vi "MATLAB.vi"(4 "Marker Style":string, 5 "Border Hit Style":string, 6 "Line Style":string, 7 "Border Win Color":u32, 8 "error in (no error)":errorcluster, 9 "Border Loss Color":u32, 10 "Ball Coordinates":cluster{"Array":dbl[], "Array 2":dbl[]}[](array[cluster]), 11 "Folder Path":path) -> (0 "error out":errorcluster, 3 "MATLAB Script":string)   [LabVIEW 2023]
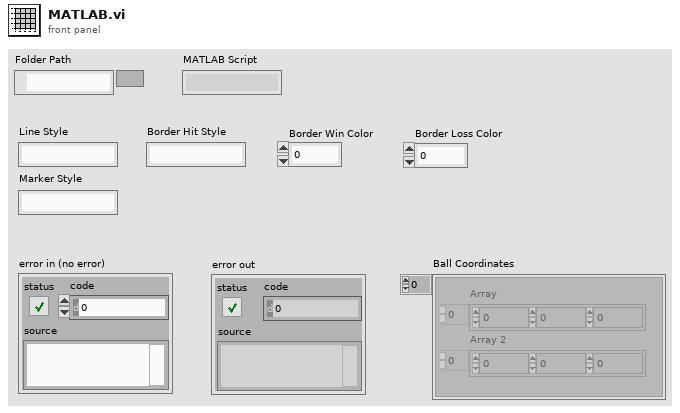
[diagram p1: front panel]
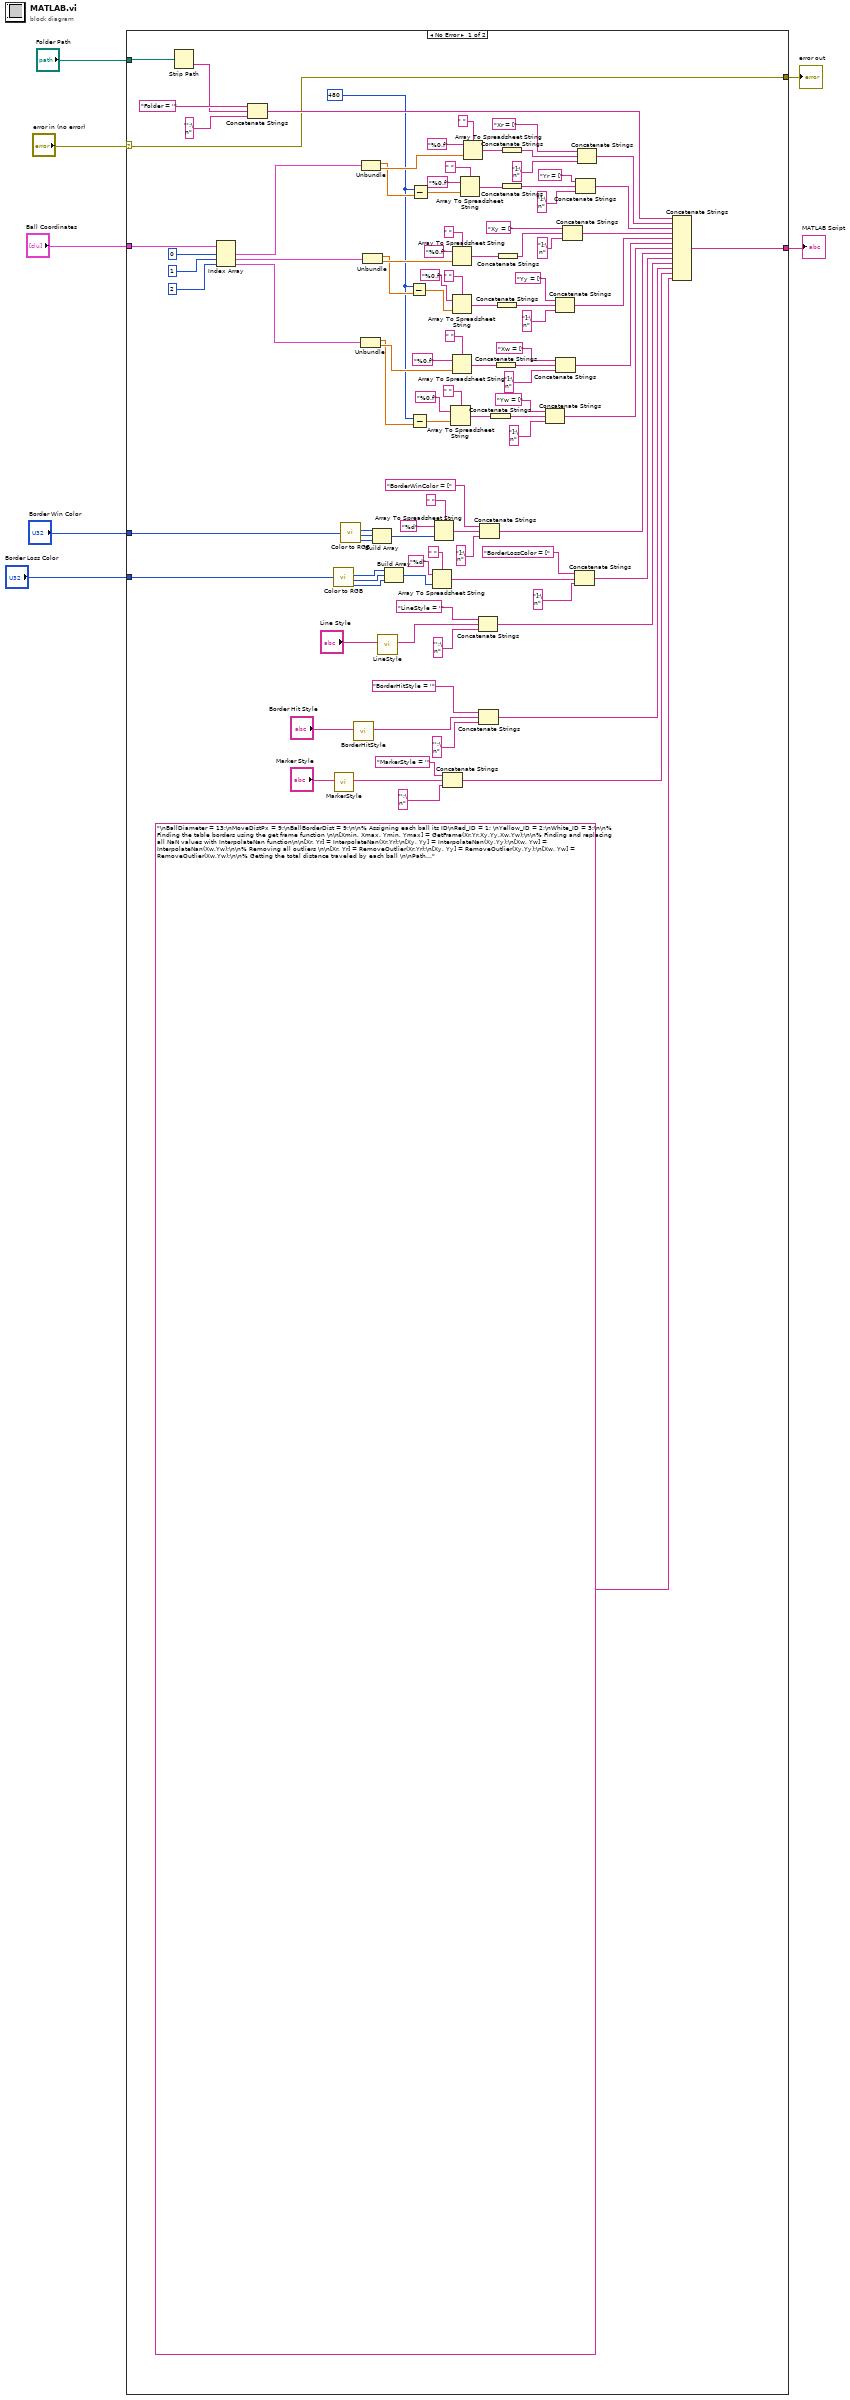
[diagram p0: block diagram]
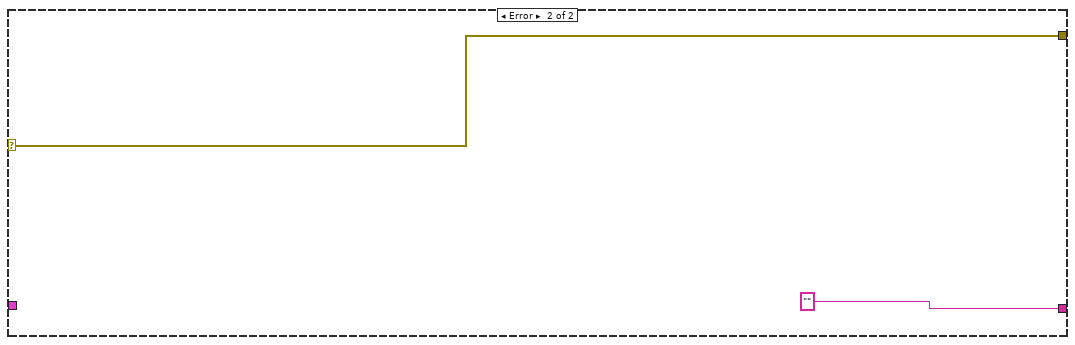
[diagram p2: hidden frame]
diagram:
  n1 = case shown="No Error" "error in (no error)" {
    selector: "error in (no error)" -> [w27 w113]
    tunnel: "Folder Path" -> [w111 _]
    tunnel: "Ball Coordinates" -> [w106 _]
    tunnel: "Border Win Color" -> [w48 _]
    tunnel: [w27 w113] -> w3
    tunnel: [w35 ""] -> w2
    tunnel: "Border Loss Color" -> [w26 _]
    frame No Error {
      w28 = 480
      n2 = Strip Path(path=w111) -> (name=w108:string)  [unwired: 1 out]
      n3 = Index Array(array=w106, index #1=0, index #2=1, index #3=2) -> (element #1=w102:cluster{"Array":dbl[], "Array 2":dbl[]}, element #2=w101:cluster{"Array":dbl[], "Array 2":dbl[]}, element #3=w100:cluster{"Array":dbl[], "Array 2":dbl[]})
      n4 = Concatenate Strings("Folder = '", w108, "';\n") -> (w107:string)
      n5 = call <vilib>:"Color to RGB.vi"("Color"=w26) -> ("R"=w25:u8, "G"=w24:u8, "B"=w23:u8)  [unwired: 1 out]
      n6 = call "MarkerStyle.vi"("Marker Style"="Marker Style") -> ("Used Marker Style"=w12:string)  [unwired: 10 in]
      n7 = call <vilib>:"Color to RGB.vi"("Color"=w48) -> ("R"=w47:u8, "G"=w46:u8, "B"=w45:u8)  [unwired: 1 out]
      n8 = call "BorderHitStyle.vi"("Border Hit Style"="Border Hit Style") -> ("Used Border Hit Style"=w29:string)  [unwired: 10 in]
      n9 = Unbundle(w100) -> ("Array"=w57:dbl[], "Array 2"=w65:dbl[])
      n10 = Unbundle(w102) -> ("Array"=w91:dbl[], "Array 2"=w97:dbl[])
      n11 = Unbundle(w101) -> ("Array"=w75:dbl[], "Array 2"=w82:dbl[])
      n12 = Build Array(w47, w46, w45) -> (w44:u8[])
      n13 = call "LineStyle.vi"("Line Style"="Line Style") -> ("Used Line Style"=w31:string)  [unwired: 10 in]
      n14 = Build Array(w25, w24, w23) -> (w22:u8[])
      n15 = Subtract(x=w28, y=w75) -> (x-y=w73:dbl[])
      n16 = Subtract(x=w28, y=w57) -> (x-y=w56:dbl[])
      n17 = Subtract(x=w28, y=w91) -> (x-y=w90:dbl[])
      n18 = Array To Spreadsheet String(delimiter (Tab)=" ", array=w22, 3:"%d") -> (spreadsheet string=w19:string)
      n19 = Array To Spreadsheet String(delimiter (Tab)=" ", array=w44, 3:"%d") -> (spreadsheet string=w42:string)
      n20 = Concatenate Strings("MarkerStyle = '", w12, "';\n") -> (w9:string)
      n21 = Array To Spreadsheet String(delimiter (Tab)=" ", array=w56, 3:"%0.f") -> (spreadsheet string=w53:string)
      n22 = Array To Spreadsheet String(delimiter (Tab)=" ", array=w82, 3:"%0.f") -> (spreadsheet string=w74:string)
      n23 = Array To Spreadsheet String(delimiter (Tab)=" ", array=w73, 3:"%0.f") -> (spreadsheet string=w70:string)
      n24 = Array To Spreadsheet String(delimiter (Tab)=" ", array=w65, 3:"%0.f") -> (spreadsheet string=w62:string)
      n25 = Array To Spreadsheet String(delimiter (Tab)=" ", array=w90, 3:"%0.f") -> (spreadsheet string=w87:string)
      n26 = Array To Spreadsheet String(delimiter (Tab)=" ", array=w97, 3:"%0.f") -> (spreadsheet string=w95:string)
      n27 = Concatenate Strings("LineStyle = '", w31, "';\n") -> (w15:string)
      n28 = Concatenate Strings("BorderHitStyle = '", w29, "';\n") -> (w14:string)
      n29 = Concatenate Strings("BorderWinColor = [", w42, "];\n") -> (w38:string)
      n30 = Concatenate Strings(w53) -> (w52:string)
      n31 = Concatenate Strings(w62) -> (w60:string)
      n32 = Concatenate Strings(w70) -> (w69:string)
      n33 = Concatenate Strings(w74) -> (w79:string)
      n34 = Concatenate Strings(w95) -> (w94:string)
      n35 = Concatenate Strings(w87) -> (w86:string)
      n36 = Concatenate Strings("Yw = [", w52, "];\n") -> (w49:string)
      n37 = Concatenate Strings("Yy = [", w69, "];\n") -> (w66:string)
      n38 = Concatenate Strings("Xw = [", w60, "];\n") -> (w58:string)
      n39 = Concatenate Strings("Xy = [", w79, "];\n") -> (w76:string)
      n40 = Concatenate Strings("BorderLossColor = [", w19, "];\n") -> (w16:string)
      n41 = Concatenate Strings("Yr = [", w86, "];\n") -> (w83:string)
      n42 = Concatenate Strings("Xr = [", w94, "];\n") -> (w92:string)
      n43 = Concatenate Strings(w107, w92, w83, w76, w66, w58, w49, w38, w16, w15, w14, w9, "\nBallDiameter = 13;\nMoveDistPx = 9;\nBallBorderDist = 9;\n\n% Assigning each ball its ID\nRed_ID = 1; \nYellow_ID = 2;\nWhite_ID = 3;\n\n% Finding the table borders using the get frame function \n\n[Xmin, Xmax, Ymin, Ymax] = GetFrame(Xr,Yr,Xy,Yy,Xw,Yw);\n\n% Finding and replacing all NaN values with InterpolateNan function\n\n[Xr, Yr] = InterpolateNan(Xr,Yr);\n[Xy, Yy] = InterpolateNan(Xy,Yy);\n[Xw, Yw] = InterpolateNan(Xw,Yw);\n\n% Removing all outliers \n\n[Xr, Yr] = RemoveOutlier(Xr,Yr);\n[Xy, Yy] = RemoveOutlier(Xy,Yy);\n[Xw, Yw] = RemoveOutlier(Xw,Yw);\n\n% Getting the total distance traveled by each ball \n\nPathLength_Red = GetBallPathLength(Xr,Yr);\nPathLength_Yellow = GetBallPathLength(Xy,Yy);\nPathLength_White = GetBallPathLength(Xw,Yw);\n\n% Getting the ball move order \n\n[FirstBall, SecondBall, LastBall, NbBallsMoved] = GetBallMoveOrder(Xr,Yr,Xy,Yy,Xw,Yw,MoveDistPx);\n\n% Assigning which ball was hit first\n\nif (FirstBall == Red_ID)\n\n    IdxTouch = GetTouchIdx(Xr,Yr,Xmin,Xmax,Ymin,Ymax,BallBorderDist);\n    X1 = Xr;\n    Y1 = Yr;\n    Color = 'Red';\n\nelseif (FirstBall == Yellow_ID)\n\n        IdxTouch = GetTouchIdx(Xy,Yy,Xmin,Xmax,Ymin,Ymax,BallBorderDist);\n        X1 = Xy;\n        Y1 = Yy;\n        Color = 'Yellow';\n\nelseif (FirstBall == White_ID)\n\n    IdxTouch = GetTouchIdx(Xw,Yw,Xmin,Xmax,Ymin,Ymax,BallBorderDist);\n    X1 = Xw;\n    Y1 = Yw;\n    Color = 'White';\n\nend\n\n% Assigning which ball was hit second\n\nif (SecondBall == Red_ID)\n    X2 = Xr;\n    Y2 = Yr;\n    SecondTouch = GetFirstMoveIdx(Xr,Yr,MoveDistPx);\nelseif (SecondBall == Yellow_ID)\n    X2 = Yy;\n    Y2 = Yy;\n    SecondTouch = GetFirstMoveIdx(Xy,Yy,MoveDistPx);\nelseif (SecondBall == White_ID)\n    X2 = Xw;\n    Y2 = Yw;\n    SecondTouch = GetFirstMoveIdx(Xw,Yw,MoveDistPx);\nend\n\n% Assigning which ball was hit last\n\nif (LastBall == Red_ID)\n    X3 = Xr;\n    Y3 = Yr;\nelseif (LastBall == Yellow_ID)\n    X3 = Xy;\n    Y3 = Yy;\nelseif (LastBall == White_ID)\n    X3 = Xw;\n    Y3 = Yw;\nend\n\nIdxTouch = IdxTouch(IdxTouch >= SecondTouch); % Taking border touches only after the second ball is hit\nBorderHits = length(IdxTouch); % Counting border hits\nNbBallsMoved = NbBallsMoved; % Number of balls moved\n\n% Win or loss ? \n\nif NbBallsMoved == 3 && BorderHits >= 3\n    Result = 'Win';\n    BorderHitColor = BorderWinColor/255;\nelse\n    Result = 'Loss';\n    BorderHitColor = BorderLossColor/255;\nend\n\n% Creating score sheet\n\nfigure('Name','ScoreSheet','NumberTitle','off')\nhold all\n\nset(gcf,'color','white')\naxis([Xmin Xmax 0 Ymax])\naxis off\n\n% Creating rectangle representing the frame\n\nrectangle('Position',[Xmin Ymin Xmax-Xmin Ymax-Ymin],'EdgeColor','b','LineWidth',1)\n\n% Plotting ball trajectories\n\nplot(Xr,Yr,[LineStyle, 'r'],'Marker',MarkerStyle,'MarkerFaceColor','r')\nplot(Xy,Yy,[LineStyle, 'y'],'Marker',MarkerStyle,'MarkerFaceColor','y')\nplot(Xw,Yw,[LineStyle, 'b'],'Marker',MarkerStyle,'MarkerFaceColor','b')\n\n% Plotting the first position of each ball\n\nplot(Xr(1),Yr(1),'Marker','hexagram','MarkerSize',15,'MarkerEdgeColor','r')\nplot(Xy(1),Yy(1),'Marker','hexagram','MarkerSize',15,'MarkerEdgeColor','y')\nplot(Xw(1),Yw(1),'Marker','hexagram','MarkerSize',15,'MarkerEdgeColor','b')\n\n% Plotting the border hits using the chosen BorderHitStyle and\n% BorderHitColor from LabVIEW\n\nscatter(X1(IdxTouch),Y1(IdxTouch),100,'Marker',BorderHitStyle,'MarkerEdgeColor',BorderHitColor)\n\n% Displaying the captions of the score-sheet\n\nt = char(datetime('now'));\ntitle(['Score Sheet - ' Folder ' - (' t ')'],'FontSize',15);\n\ntext(Xmin + (Xmax - Xmin)*0.125,Ymin*0.75,{['Score sheet for ' '\"' Color ' Ball' '\"'],['--- ' Result ' ---']});\n\ntext(Xmin + (Xmax - Xmin)*0.125,Ymin*0.25,['dist(R):' num2str(int32(PathLength_Red)) 'px']);\ntext(Xmin + (Xmax - Xmin)*0.375,Ymin*0.25,['dist(Y):' num2str(int32(PathLength_Yellow)) 'px']);\ntext(Xmin + (Xmax - Xmin)*0.625,Ymin*0.25,['dist(W):' num2str(int32(PathLength_White)) 'px']);\n\ntext(Xmin + (Xmax - Xmin)*0.625,Ymin*0.75,{[num2str(NbBallsMoved) ' ball(s) touched'],[num2str(BorderHits) ' band(s) touched']}) \n\nhold off \n\n% Saving the score-sheet as a .pdf file under the format ScoreSheetTx.pdf\n\nfilename = sprintf('ScoreSheet%s',Folder);\nsaveas(gcf,filename,'pdf');\n\n%% AnalyseTx.m \n% \n% Authors:\n%   Roy Turk 34 55 77\n%   Selim Sherif 34 60 35\n%\n% Script containing a combination of functions that will receive the ball \n% coordinates from LabVIEW and display the score-sheet with the final \n% result of the game.") -> (w35:string)
    }
    frame Error {
    }
  }
  "MATLAB Script" <- w2
  "error out" <- w3
